vi "AgentMsgCreator.vi"(5 "tp":string, 6 "dt":string, 7 "id":string, 8 "ct":dbl=-1.0, 9 "rp":dbl=-1.0, 10 "rq":dbl, 11 "cmd":string) -> (2 "JSON字符串":string)   [LabVIEW 2016]
panel:
  # "设备ID"
  # "Type，设备类型"
  # "command，命令类型"
  # "requestId，上层发出的控制命令id"
  # "responseId，底层发回的反馈id，结合requestId表明是对reqId的第几次反馈"
  # "计算时间，此处忽略"
  # "实际传输的数据"
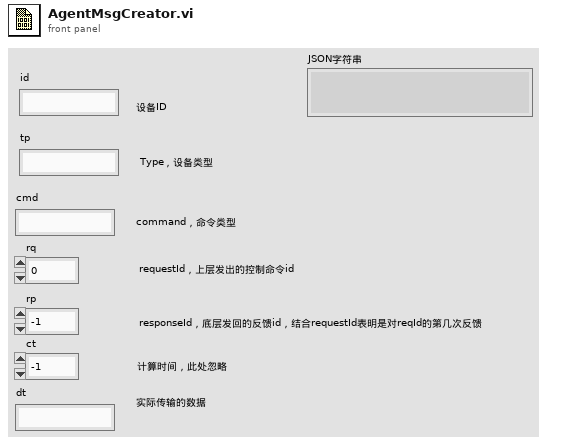
[diagram p1: front panel]
types:
  T1 = cluster{"id":string, "tp":string, "cmd":string, "rq":dbl, "rp":dbl, "ct":dbl, "dt":string}
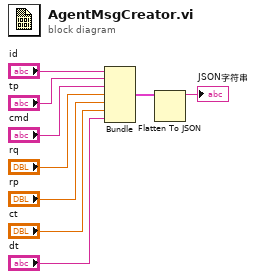
[diagram p0: block diagram]
diagram:
  n1 = Bundle("id"="id", "tp"="tp", "cmd"="cmd", "rq"="rq", "rp"="rp", "ct"="ct", "dt"="dt") -> (w1:T1)  [unwired: 1 in]
  n2 = Flatten To JSON(anything=w1) -> (JSON string=→"JSON字符串":string)  [unwired: 2 in, 1 out]
